vi "Write Listening TS.vi"(8 "error in (no error)":errorcluster, 10 "Listening":u64, 11 "CIFCorePlugin in":refnum<class "CIFCorePlugin.lvclass">) -> (0 "error out":errorcluster, 3 "CIFCorePlugin out":refnum<class "CIFCorePlugin.lvclass">)   [LabVIEW 2021, in "CIFCorePlugin.lvclass"]
doc: "Update the timestamp. Time is U64, absolute time in nS in the appropriate clockID configured for the plugin. If a 0 is wired it will automatically get the current time."
uses:
  CIFCorePlugin.lvclass
  CIFCorePlugin.lvclass/CIFCorePlugin.ctl
  CIFUtilities/CIFClocks/Time Conversion/LabVIEW Time to UTC Time.vi
  Common/Utilities/Add Error.vi
  Common/Utilities/Append Error Location.vi
  <vilib>/CIF Foundation/CIF Utilities/Time/Time_CIF_U.lvlib
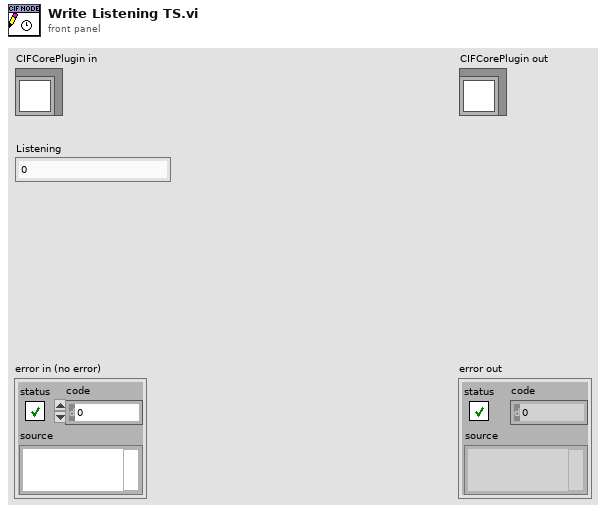
[diagram p1: front panel]
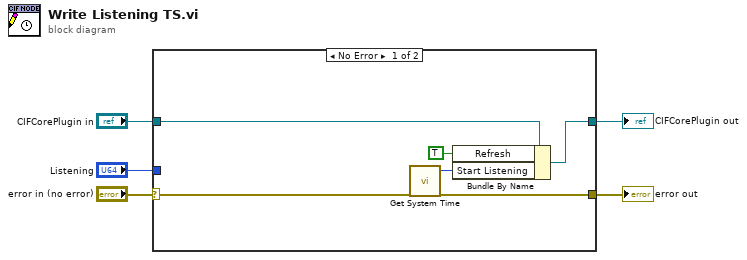
[diagram p0: block diagram]
diagram:
  n1 = case shown="No Error" "error in (no error)" {
    selector: "error in (no error)" -> [w6 w11]
    tunnel: [w6 w11] -> w4
    tunnel: [w10 w12] -> w2
    tunnel: "CIFCorePlugin in" -> [w7 w12]
    tunnel: "Listening" -> [_ _]
    frame No Error {
      n2 = call <vilib>:"Get System Time.vi"() -> ("Time (ns)"=w8:i64)  [unwired: 5 in]
      n3 = Bundle By Name(cluster=w7, "Refresh"=TRUE, "Start Listening"=w8) -> (w10:refnum<class "CIFCorePlugin.lvclass">)
    }
    frame Error {
    }
  }
  "error out" <- w4
  "CIFCorePlugin out" <- w2
